vi "Cowl_Set.vi"   [LabVIEW 2020]
uses:
  Globals/Cowl_Globals.vi
  Cowl_States.ctl
  Cowl_Cluster.ctl
types:
  T1 = typedef "Cowl_Cluster.ctl" = cluster{"Control_State\n":T2, "Manual_Cowl_%Power":dbl}
  T2 = typedef "Cowl_States.ctl" = enum16{"Manual_%VBus", "GoToAngle"}
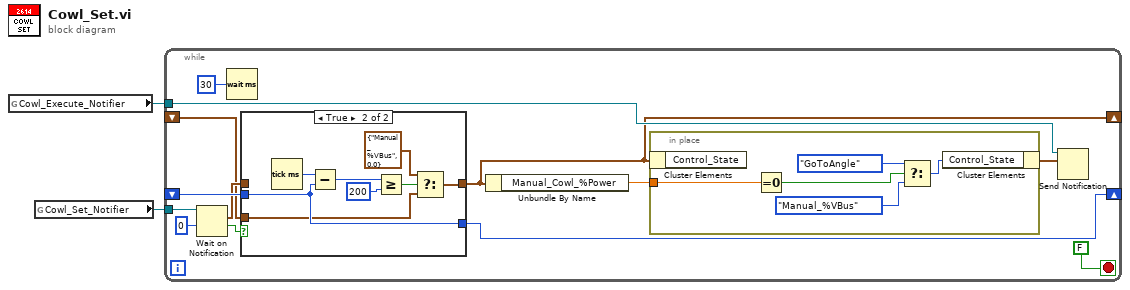
[diagram p0: block diagram]
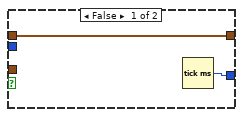
[diagram p2: hidden frame]
diagram:
  n1 = global read "Cowl_Globals.vi" "Cowl_Execute_Notifier"() -> (w2:refnum<notifier>)
  n2 = global read "Cowl_Globals.vi" "Cowl_Set_Notifier"() -> (w1:refnum<notifier>)
  n3 = while {
    tunnel: w2 -> [w13]
    tunnel: w1 -> [w12]
    shift-right: [w8] -> _
    shift-left: _ -> [w9]
    shift-right: [w6] -> _
    shift-left: _ -> [w4]
    stop <- FALSE stop-if-true
    n4 = Wait on Notification(notifier=w12, timeout in ms (-1)=0) -> (notification=w5:T1, timed out?=w7:bool)  [unwired: 2 in, 2 out]
    n5 = Wait (ms)(milliseconds to wait=u32 30) -> ()  [unwired: 1 out]
    n6 = case shown="True" w7 {
      tunnel: w5 -> [w17 _]
      tunnel: [w17 w20] -> w6
      tunnel: [w16 w24] -> w8
      tunnel: w9 -> [_ w24]
      tunnel: w4 -> [_ w19]
      frame False {
        n7 = Tick Count (ms)() -> (millisecond timer value=w16:u32)
      }
      frame True {
        n8 = Tick Count (ms)() -> (millisecond timer value=w25:u32)
        n9 = Subtract(x=w25, y=w24) -> (x-y=w23:u32)
        n10 = Greater Or Equal?(x=w23, y=u32 200) -> (x >= y?=w21:bool)
        n11 = Select(t=T1 {"Control_State\n"=enum."Manual_%VBus", "Manual_Cowl_%Power"=0.0} ("notification"), s=w21, f=w19) -> (s? t:f=w20:T1)
      }
    }
    n12 = Unbundle By Name(w6) -> ("Manual_Cowl_%Power"=w11:dbl)
    n13 = in-place {
      in-place-border: w11 -> [w30]
      n14 = in-place-cluster #1(w6) -> ()  [unwired: 1 out]
      n15 = Equal To 0?(x=w30) -> (x = 0?=w28:bool)
      n16 = Select(t=Cowl_States."GoToAngle" ("Control_State"), s=w28, f=Cowl_States."Manual_%VBus" ("Control_State")) -> (s? t:f=w29:T2)
      n17 = in-place-cluster #1("Control_State"=w29) -> (w10:T1)
    }
    n18 = Send Notification(notification=w10, notifier=w13) -> ()  [unwired: 1 in, 2 out]
  }
